vi "Engine Simulation Main Page.vi"(8 "error in (no error)":errorcluster, 11 "Node Ptr":T1 format="%.0x") -> (0 "error out":errorcluster)   [LabVIEW 2011, in "Engine Sim System Explorer.lvlib"]
uses:
  Engine Sim System Explorer.lvlib
  <vilib>/NI Veristand/Custom Device API/Custom Device Item Ref.ctl
  <vilib>/NI Veristand/Custom Device API/Get Item Property (Boolean).vi
  Shared/Engine Simulation Global.vi
  <vilib>/NI Veristand/Custom Device API/Get Item Property (String).vi
  <vilib>/NI Veristand/Custom Device API/Set Item Property (String).vi
  <vilib>/NI Veristand/Custom Device API/Custom Device API.lvlib
  Engine Simulation Shared.lvlib
panel:
  out "Version":string
  in  "FPGA Addr Ctl":string caption="FPGA Address"
  in  "SHDocVw.IWebBrowser2":refnum<k7>(container)
  out "FPGA Address":string
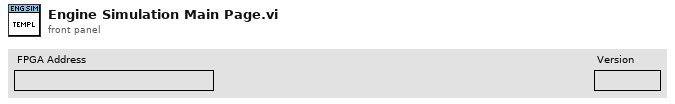
[diagram p1: front panel]
types:
  T1 = typedef "Custom Device API.lvlib/Custom Device Item Ref.ctl" = u64
  T2 = typedef "Custom Device API.lvlib/Custom Device Commands.ctl" = enum16{"Default", "Item renamed", "Shutdown", "Dynamic button pressed"}
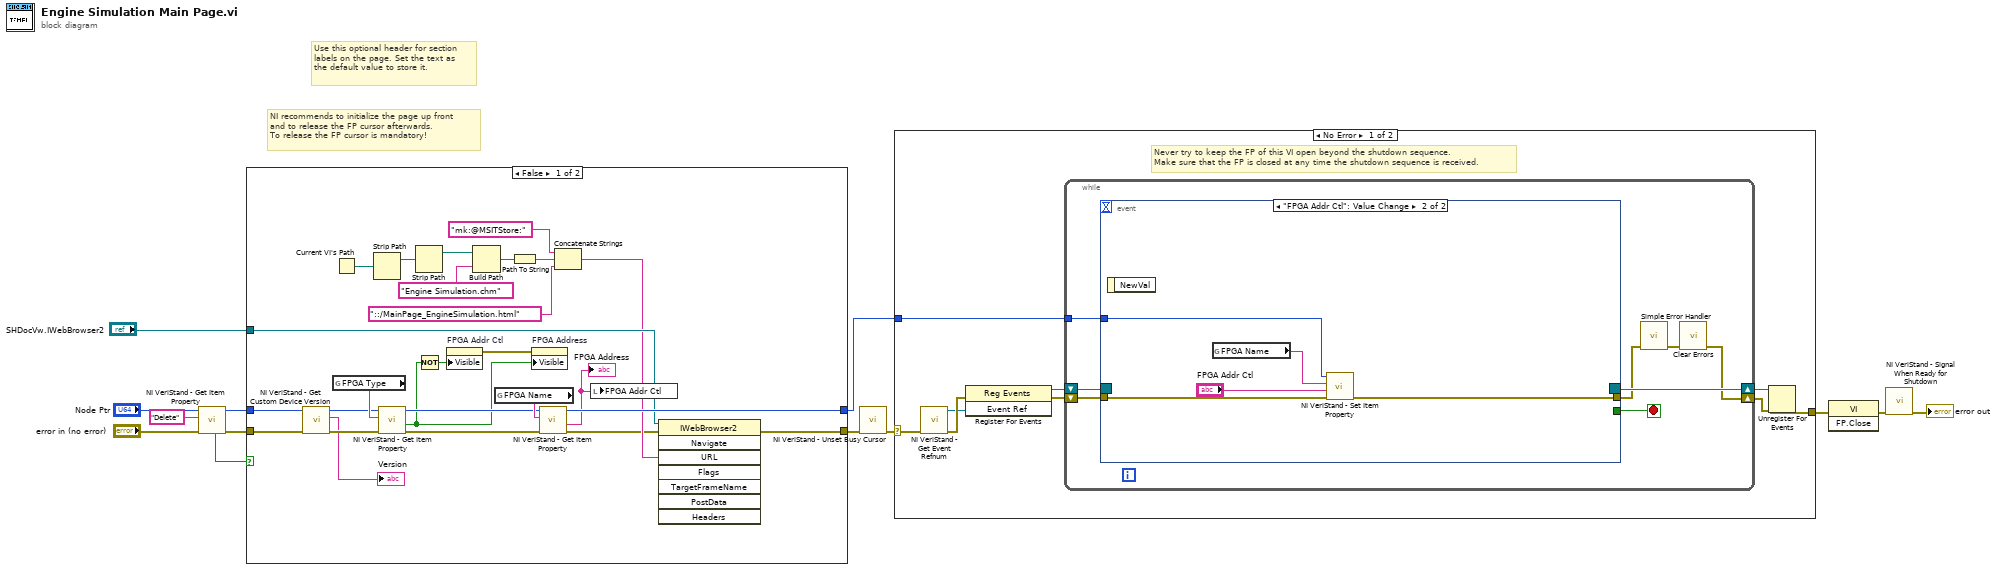
[diagram p0: block diagram]
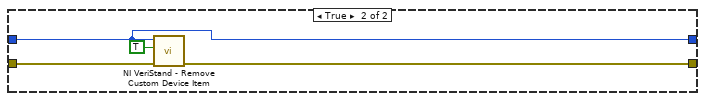
[diagram p2: hidden frame]
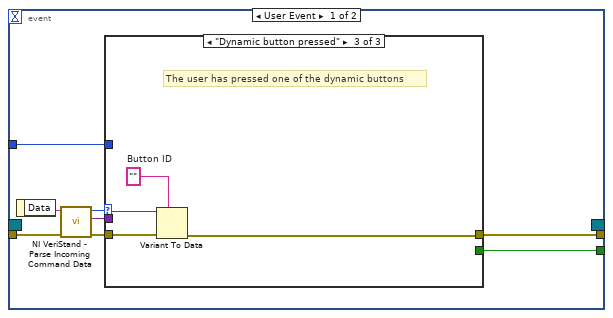
[diagram p3: hidden frame]
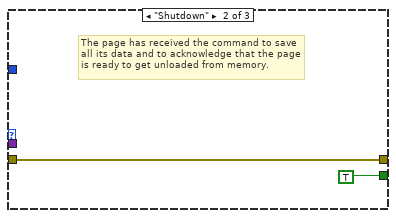
[diagram p5: hidden frame]
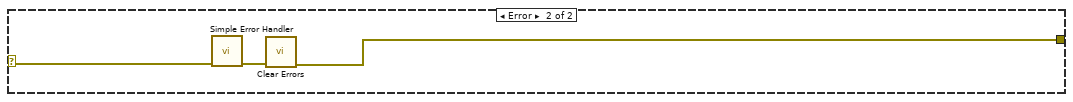
[diagram p6: hidden frame]
diagram:
  # "Use this optional header for section labels on the page. Set the text as the default value to store it."
  # "NI recommends to initialize the page up front\nand to release the FP cursor afterwards.\nTo release the FP cursor is mandatory!"
  n1 = call-poly <vilib>:"NI VeriStand - Get Item Property.vi"("error in (no error)"="error in (no error)", "Property Name"="Delete", "Item Ref in"="Node Ptr") -> ("error out"=w4:errorcluster, "Item Ref out"=w3:T1, "Found?"=w1:bool)  [unwired: 5 in, 1 out]
  n2 = case shown="False" w1 {
    tunnel: [w39 w42] -> w10
    tunnel: [w38 w41] -> w8
    tunnel: "SHDocVw.IWebBrowser2" -> [w37 _]
    tunnel: w4 -> [w36 w43]
    tunnel: w3 -> [w16 w41]
    frame False {
      n3 = call <vilib>:"NI VeriStand - Get Custom Device Version.vi"("error in (no error)"=w36, "Device Ref in"=w16) -> ("error out"=w17:errorcluster, "Value"=→"Version":string, "Device Ref out"=w15:T1)  [unwired: 7 in]
      n4 = global read "Engine Simulation Global.vi" "FPGA Type"() -> (w24:string)
      n5 = Current VI's Path() -> (path=w33:path)
      n6 = Strip Path(path=w33) -> (stripped path=w32:path)  [unwired: 1 out]
      n7 = call-poly <vilib>:"NI VeriStand - Get Item Property.vi"("error in (no error)"=w17, "Property Name"=w24, "Item Ref in"=w15) -> ("error out"=w23:errorcluster, "Value"=w19:bool, "Item Ref out"=w22:T1)  [unwired: 5 in, 1 out]
      n8 = Strip Path(path=w32) -> (stripped path=w27:path)  [unwired: 1 out]
      n9 = Not(x=w19) -> (.not. x?=w20:bool)
      n10 = property on="FPGA Addr Ctl" class="Str"("Visible"=w20) -> (error out=w21:errorcluster)  [unwired: 2 in, 1 out]
      n11 = Build Path(base path=w27, name or relative path="Engine Simulation.chm") -> (appended path=w29:path)
      n12 = global read "Engine Simulation Global.vi" "FPGA Name"() -> (w35:string)
      n13 = Path To String(path=w29) -> (string=w30:string)
      n14 = property on="FPGA Address" class="Str"(error in=w21, "Visible"=w19) -> ()  [unwired: 1 in, 2 out]
      n15 = call-poly <vilib>:"NI VeriStand - Get Item Property.vi"("error in (no error)"=w23, "Property Name"=w35, "Item Ref in"=w22) -> ("error out"=w18:errorcluster, "Value"=w25:string, "Item Ref out"=w38:T1)  [unwired: 5 in, 1 out]
      "FPGA Address" <- w25
      n16 = Concatenate Strings("mk:@MSITStore:" ("string"), w30, "::/MainPage_EngineSimulation.html" ("name or relative path")) -> (w26:string)
      n17 = local write "FPGA Addr Ctl"(w25) -> ()
      n18 = invoke class="IWebBrowser2" method="Navigate"(reference=w37, error in=w18, "URL"=w26) -> (error out=w39:errorcluster)  [unwired: 5 in, 7 out]
    }
    frame True {
      n19 = call <vilib>:"NI VeriStand - Remove Custom Device Item.vi"("error in (no error)"=w43, "Force Delete (F)"=TRUE, "Item Ref in"=w41) -> ("error out"=w42:errorcluster)  [unwired: 7 in, 1 out]
    }
  }
  n20 = call <vilib>:"NI VeriStand - Unset Busy Cursor.vi"("error in (no error)"=w10) -> ("error out"=w9:errorcluster)  [unwired: 10 out]
  n21 = case shown="No Error" w9 {
    selector: w9 -> [w44 w83]
    tunnel: [w49 w81] -> w13
    tunnel: w8 -> [w45 _]
    frame No Error {
      # "Never try to keep the FP of this VI open beyond the shutdown sequence.\nMake sure that the FP is closed at any time the shutdown sequence is received."
      n22 = call <vilib>:"NI VeriStand - Get Event Refnum.vi"("error in (no error)"=w44) -> ("error out"=w52:errorcluster, "Event Ref"=w48:refnum<user-event>)  [unwired: 9 out]
      n23 = register-events(error in=w52, w48) -> (reference out=w46:refnum<event-registration>, error out=w47:errorcluster)  [unwired: 1 in]
      n24 = while {
        tunnel: w45 -> [w56]
        shift-right: [w53] -> w50
        shift-left: w47 -> [w59]
        shift-right: [w60] -> w51
        shift-left: w46 -> [w58]
        stop <- w57 stop-if-true
        n25 = event shown="[1] \"FPGA Addr Ctl\": Value Change" {
          selector: w58 -> [_ _]
          dyn-events: [_ _] -> w60
          timeout: _ -> [_ _]
          tunnel: w59 -> [w68 w80]
          tunnel: [w64 _] -> w57
          tunnel: [w63 w79] -> w55
          tunnel: w56 -> [w62 w78]
          event User Event {
            n26 = event-data() -> ("Data"=w67:string)  [unwired: 1 out]
            n27 = call <vilib>:"NI VeriStand - Parse Incoming Command Data.vi"("error in (no error)"=w68, "Incoming data"=w67) -> ("error out"=w66:errorcluster, "Outgoing data"=w61:variant, "Action"=w65:T2)  [unwired: 7 out]
            n28 = case shown="\"Dynamic button pressed\"" w65 {
              tunnel: w66 -> [w69 w70 w75]
              tunnel: [_ TRUE _] -> w64
              tunnel: [w69 w70 w72] -> w63
              tunnel: w62 -> [_ _ _]
              tunnel: w61 -> [_ _ w74]
              frame "Default", Default {
              }
              frame "Shutdown" {
                # "The page has received the command to save all its data and to acknowledge that the page is ready to get unloaded from memory."
              }
              frame "Dynamic button pressed" {
                w73 = ""  # Button ID
                # "The user has pressed one of the dynamic buttons"
                n29 = Variant To Data(error in=w75, type=w73, Variant=w74) -> (error out=w72:errorcluster)  [unwired: 1 out]
              }
            }
          }
          event "FPGA Addr Ctl": Value Change {
            n30 = event-data() -> ()  [unwired: 2 out]
            n31 = global read "Engine Simulation Global.vi" "FPGA Name"() -> (w76:string)
            n32 = call-poly <vilib>:"NI VeriStand - Set Item Property.vi"("error in (no error)"=w80, "Value"="FPGA Addr Ctl", "Property Name"=w76, "Item Ref in"=w78) -> ("error out"=w79:errorcluster)  [unwired: 5 in, 2 out]
          }
        }
        n33 = call <vilib>:"Simple Error Handler.vi"("error in (no error)"=w55) -> ("error out"=w54:errorcluster)  [unwired: 1 in, 7 out]
        n34 = call <vilib>:"Clear Errors.vi"("error in (no error)"=w54) -> ("error out"=w53:errorcluster)  [unwired: 6 out]
      }
      n35 = Unregister For Events(event registration refnum=w51, error in=w50) -> (error out=w49:errorcluster)
    }
    frame Error {
      n36 = call <vilib>:"Simple Error Handler.vi"("error in (no error)"=w83) -> ("error out"=w82:errorcluster)  [unwired: 1 in, 7 out]
      n37 = call <vilib>:"Clear Errors.vi"("error in (no error)"=w82) -> ("error out"=w81:errorcluster)  [unwired: 6 out]
    }
  }
  n38 = invoke class="VI" method="FP.Close"(error in=w13) -> (error out=w12:errorcluster)  [unwired: 2 in, 2 out]
  n39 = call <vilib>:"NI VeriStand - Signal When Ready for Shutdown.vi"("error in (no error)"=w12) -> ("error out"=→"error out":errorcluster)  [unwired: 10 out]
